vi "HSOpMux.vi"() -> ()   [LabVIEW 2013]
uses:
  Multiplexer_Opmux.lvclass
  HS3.llb/GlobalVariables.vi
  OverallRoutines/HS3OverallRoutines.lvlib
panel:
  in  "TimeForEachScan":dbl[](array[numeric])
  out "tmr":u32 caption="Elapsed for acq"
  in  "Run":bool
  out "Channels":refnum<vi>[](array[refnum])
  out "Ch8":dbl[](graph)
  out "Ch7":dbl[](graph)
  out "Ch6":dbl[](graph)
  out "Ch5":dbl[](graph)
  out "Ch4":dbl[](graph)
  out "Ch3":dbl[](graph)
  out "Ch2":dbl[](graph)
  out "Ch1":dbl[](graph)
  in  "Scan":bool
  in  "Set":bool
  in  "Length":dbl=1.0 caption="Length (us)" min=0.1 max=6.3 step=0.1
  in  "Voltage":dbl min=0.0 max=1023.0 step=1.0
  in  "Into":u16[](array[numeric])
  in  "Forward":u16[](array[numeric])
  in  "Signal Frequency":u32(ring)=10000000 items=["5Mhz"=5000000, "10Mhz"=10000000, "25Mhz"=25000000]
  in  "Shutdown":bool
  out "Acq":bool caption="Acquiring"
  out "SampleFrequency":dbl format="%#_8g"
  out "ChArray":dbl[](array[numeric])
  out "Serial":i32
  out "DllPath":path
  out "HandyScope":bool
  out "Multiplexer":bool
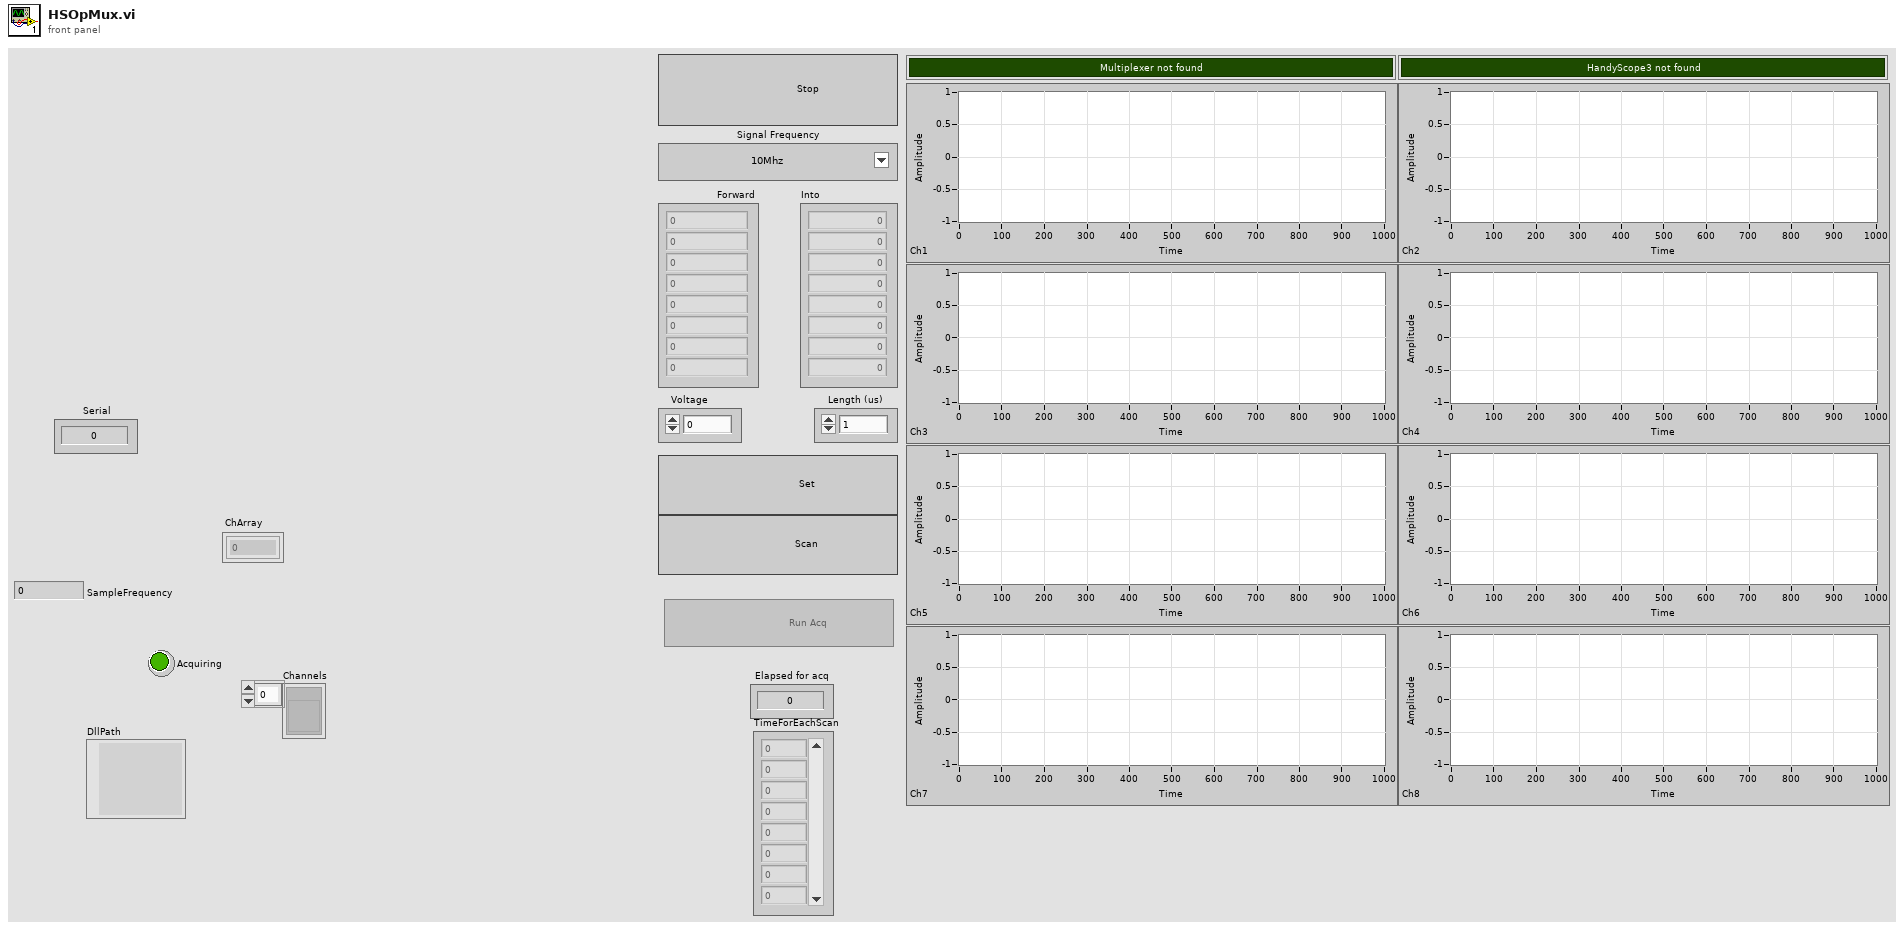
[diagram p1: front panel]
types:
  T1 = cluster{"trgSource":u16, "trgMode":u16, "trgLevel":dbl}
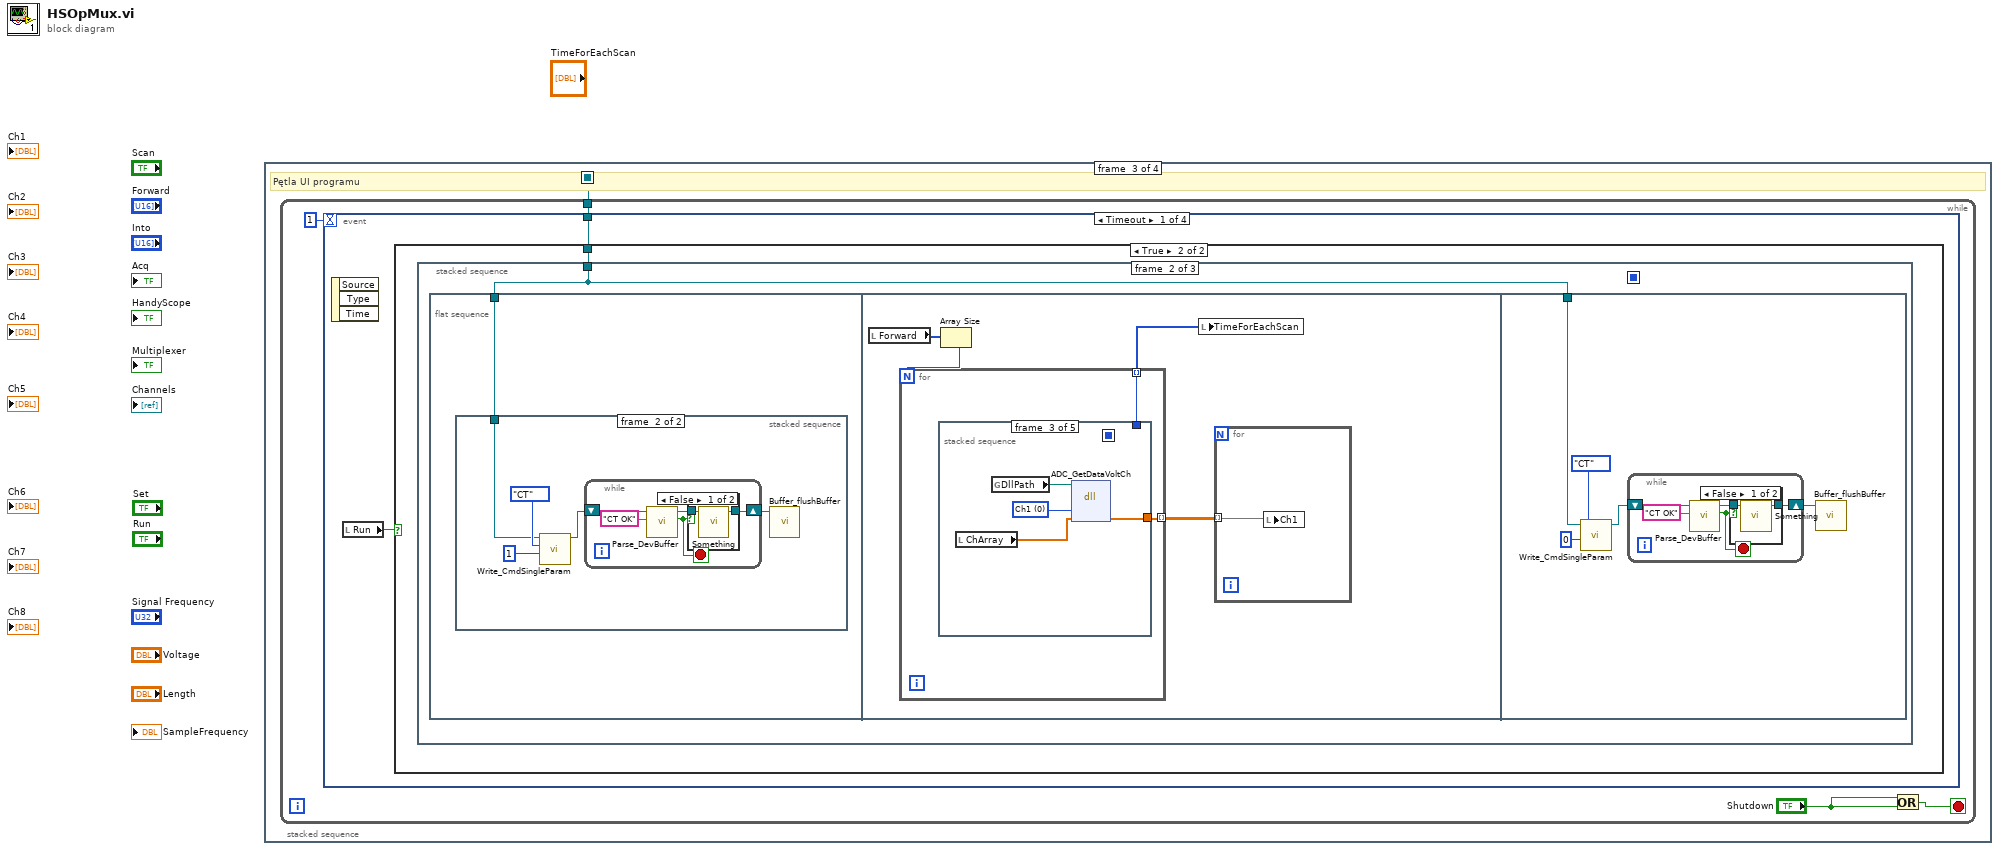
[diagram p0: block diagram]
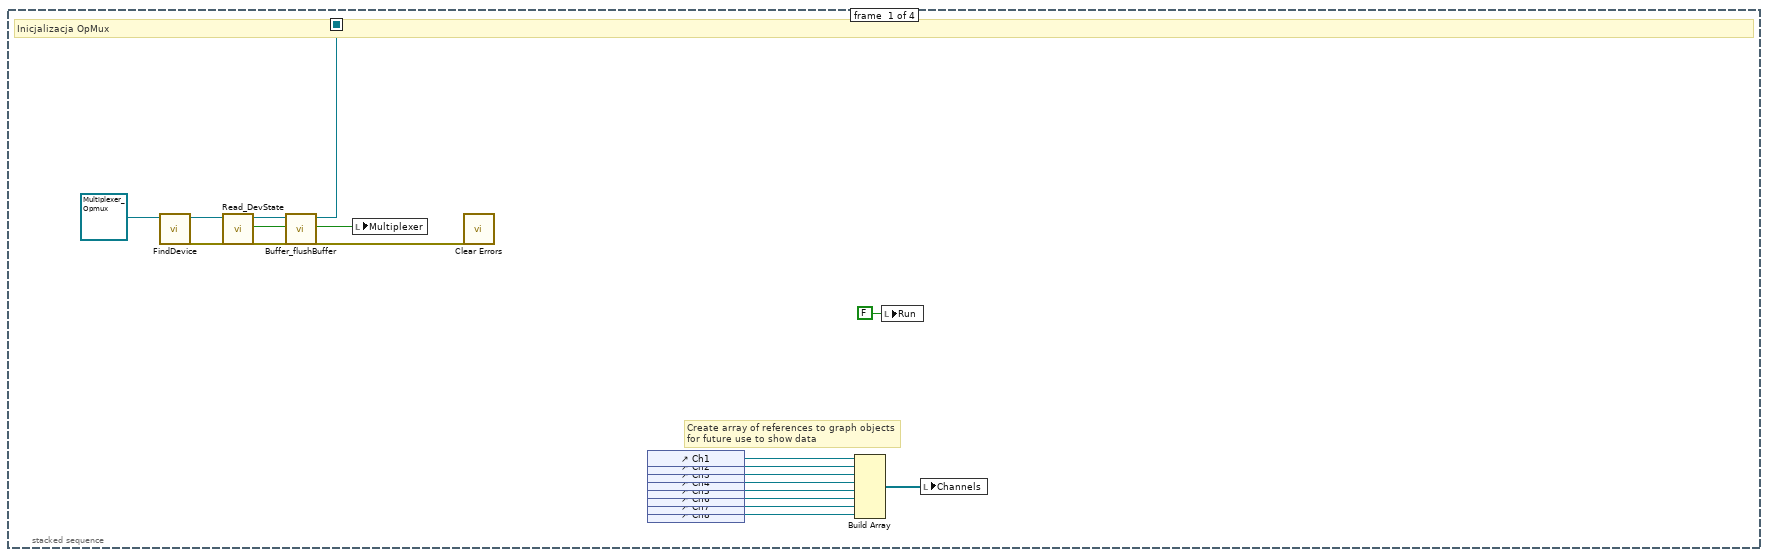
[diagram p2: hidden frame]
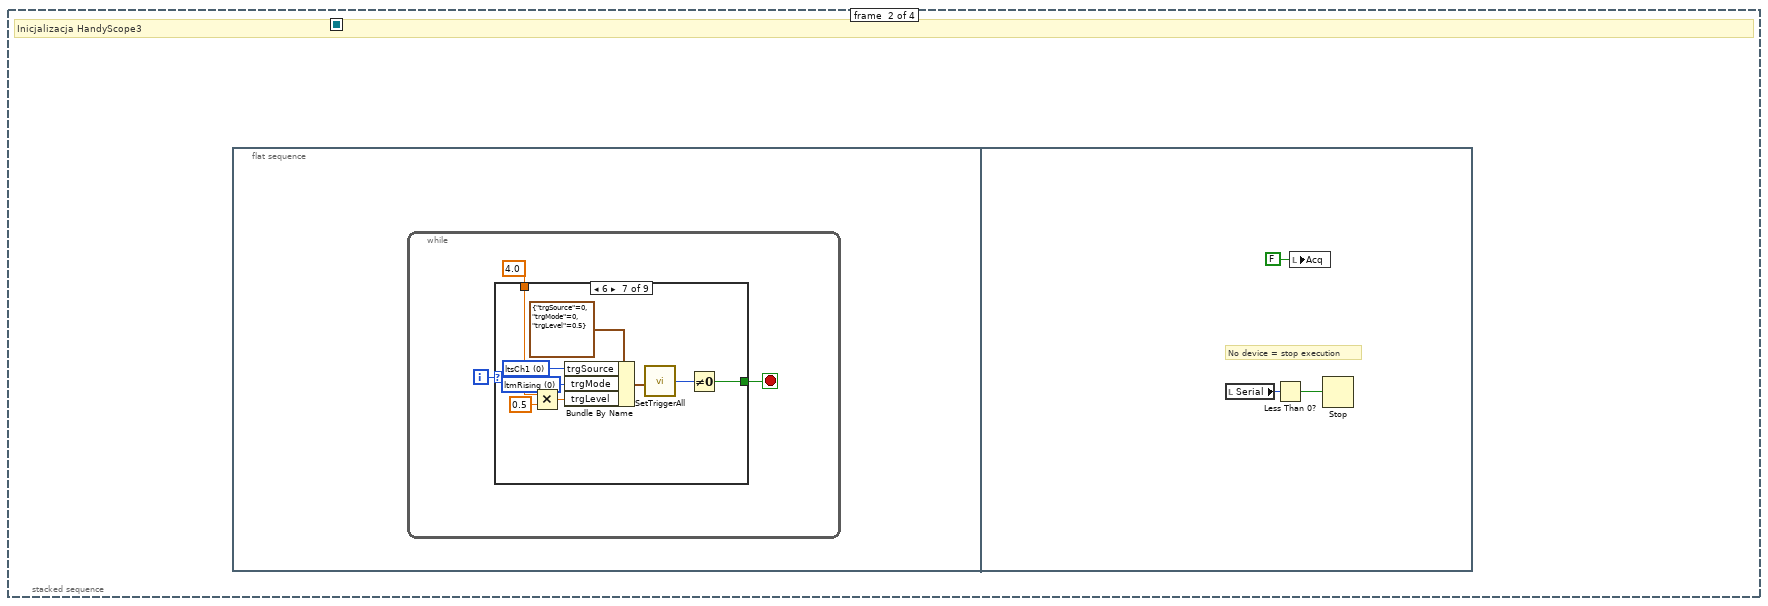
[diagram p3: hidden frame]
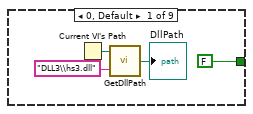
[diagram p4: hidden frame]
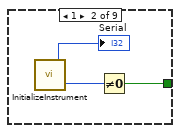
[diagram p5: hidden frame]
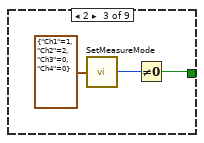
[diagram p6: hidden frame]
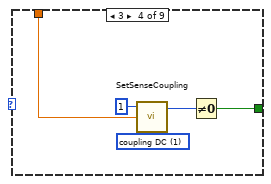
[diagram p7: hidden frame]
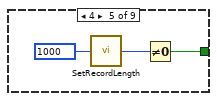
[diagram p8: hidden frame]
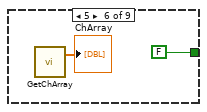
[diagram p9: hidden frame]
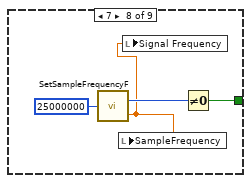
[diagram p10: hidden frame]
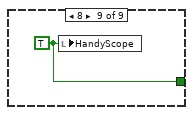
[diagram p11: hidden frame]
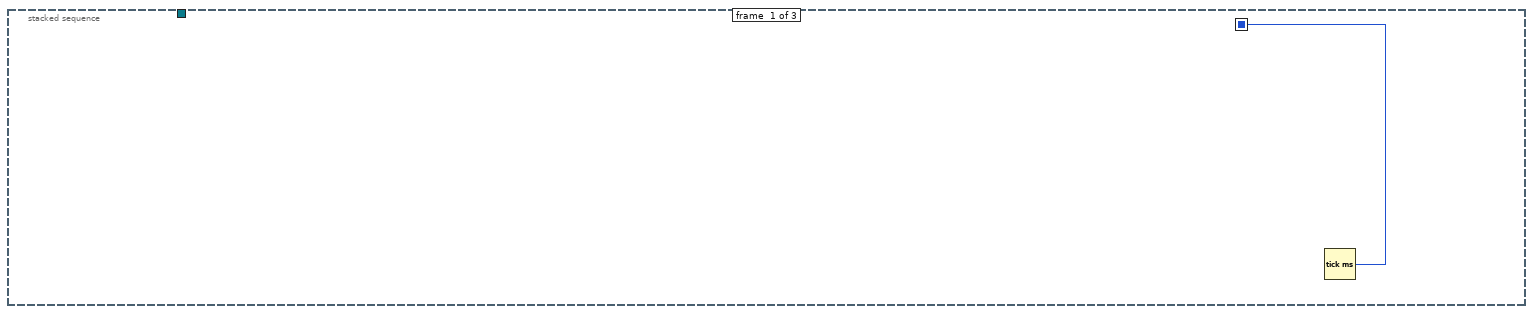
[diagram p13: hidden frame]
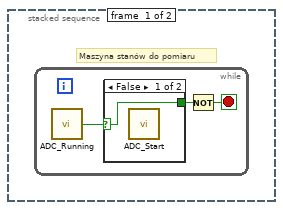
[diagram p14: hidden frame]
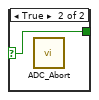
[diagram p15: hidden frame]
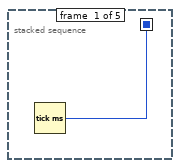
[diagram p17: hidden frame]
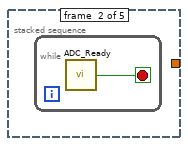
[diagram p18: hidden frame]
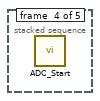
[diagram p19: hidden frame]
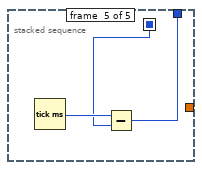
[diagram p20: hidden frame]
diagram:
  n1 = stacked-sequence {
    seq-local: [w1 _ _ _] -> [_ _ w59 _]
    frame #0 {
      # "Create array of references to graph objects\nfor future use to show data"
      # "Inicjalizacja OpMux"
      n2 = call-dynamic "FindDevice.vi"("Multiplexer_Opmux in"=refnum<class "Multiplexer_Opmux.lvclass"> refnum) -> ("error out"=w15:errorcluster, "Multiplexer_Opmux out"=w17:refnum<class "Multiplexer_Opmux.lvclass">)  [unwired: 8 in, 1 out]
      n3 = call-dynamic "Read_DevState.vi"("error in (no error)"=w15, "Multiplexer_Opmux in"=w17) -> ("error out"=w3:errorcluster, "DevState"=w16:bool, "Multiplexer_Opmux out"=w4:refnum<class "Multiplexer_Opmux.lvclass">)  [unwired: 7 in]
      n4 = call-dynamic "Buffer_flushBuffer.vi"("error in (no error)"=w3, "Multiplexer_Opmux in"=w4) -> ("error out"=w2:errorcluster, "Multiplexer_Opmux out"=w1:refnum<class "Multiplexer_Opmux.lvclass">)  [unwired: 8 in]
      n5 = local write "Multiplexer"(w16) -> ()
      n6 = call <vilib>:"Clear Errors.vi"("error in (no error)"=w2) -> ()  [unwired: 6 in, 1 out]
      n7 = control-ref of="Ch1"() -> (w14:refnum<vi>)
      n8 = control-ref of="Ch2"() -> (w13:refnum<vi>)
      n9 = control-ref of="Ch3"() -> (w12:refnum<vi>)
      n10 = control-ref of="Ch4"() -> (w11:refnum<vi>)
      n11 = control-ref of="Ch5"() -> (w10:refnum<vi>)
      n12 = control-ref of="Ch6"() -> (w9:refnum<vi>)
      n13 = control-ref of="Ch7"() -> (w8:refnum<vi>)
      n14 = control-ref of="Ch8"() -> (w7:refnum<vi>)
      n15 = Build Array(w14, w13, w12, w11, w10, w9, w8, w7) -> (w6:refnum<vi>[])
      n16 = local write "Run"(FALSE ("Run")) -> ()
      n17 = local write "Channels"(w6) -> ()
    }
    frame #1 {
      # "Inicjalizacja HandyScope3"
      n18 = flat-sequence {
        frame #0 {
          n19 = while {
            i -> [w21]
            stop <- w20 stop-if-true
            w19 = 4.0 items=["0,2"=0.2, "0,8"=0.8, "2"=2.0, "4"=4.0, "20"=20.0, "40"=40.0, "80"=80.0] ("chSense")
            n20 = case shown="6" w21 {
              tunnel: [FALSE w26 w30 w33 w38 FALSE w49 w54 w55] -> w20
              tunnel: w19 -> [_ _ _ w32 _ _ w45 _ _]
              frame 0, Default {
                n21 = Current VI's Path() -> (path=w23:path)
                n22 = call "GetDllPath.vi"("DllName"="DLL3\\hs3.dll", "path"=w23) -> ("DllPath"=→"DllPath":path)
              }
              frame 1 {
                n23 = call "InitializeInstrument.vi"() -> ("ErrorCode"=w27:i16, "Serial"=→"Serial":i32)
                n24 = Not Equal To 0?(x=w27) -> (x != 0?=w26:bool)
              }
              frame 2 {
                n25 = call "SetMeasureMode.vi"("oModeStack"=cluster{"Ch1":u8, "Ch2":u8, "Ch3":u8, "Ch4":u8} {"Ch1"=1, "Ch2"=2, "Ch3"=0, "Ch4"=0}) -> ("ErrorCode"=w29:i16)
                n26 = Not Equal To 0?(x=w29) -> (x != 0?=w30:bool)
              }
              frame 3 {
                w36 = 1 items=["coupling AC", "coupling DC"] ("chCoupling")
                n27 = call "SetSenseCoupling.vi"("chCoupling"=w36, "chSense"=w32, "chSet"=1) -> ("ErrorCode"=w34:i16)  [unwired: 1 out]
                n28 = Not Equal To 0?(x=w34) -> (x != 0?=w33:bool)
              }
              frame 4 {
                w39 = u32 1000 items=["100"=100, "250"=250, "500"=500, "1000"=1000, "2500"=2500, "5000"=5000, "10000"=10000, "25000"=25000, "50000"=50000, "100000"=100000, "131000"=131000] ("RecordLength")
                n29 = call "SetRecordLength.vi"("RecordLength"=w39) -> ("ErrorCode"=w37:i16)
                n30 = Not Equal To 0?(x=w37) -> (x != 0?=w38:bool)
              }
              frame 5 {
                n31 = call "GetChArray.vi"() -> ("ChArray"=→"ChArray":dbl[])  [unwired: 1 out]
              }
              frame 6 {
                w42 = u16 0 items=["ltmRising", "ltmFalling", "ltmInWindow", "ltmOutWindow", "ltmTVLine", "ltmTVFieldOdd", "ltmTVFieldEven"] ("trgMode")
                w43 = u16 0 items=["ltsCh1"=0, "ltsCh2"=1, "ltsExternal"=4, "ltsAnalogExt"=5, "ltsAnd"=6, "ltsOr"=7, "ltsXor"=8, "ltsNoTrig"=9, "notUsed"=10, "ltsPxiExt"=11, "ltsGenStart"=12, "ltsGenStop"=13, "ltsGenNew"=14] ("trgSource")
                n32 = Multiply(x=w45, y=0.5) -> (x*y=w46:dbl)
                n33 = Bundle By Name(cluster=T1 {"trgSource"=0, "trgMode"=0, "trgLevel"=0.5} ("TriggerSettings"), "trgSource"=w43, "trgMode"=w42, "trgLevel"=w46) -> (w47:T1)
                n34 = call "SetTriggerAll.vi"("TriggerSettings"=w47) -> ("ErrorCode"=w50:i32)
                n35 = Not Equal To 0?(x=w50) -> (x != 0?=w49:bool)
              }
              frame 7 {
                n36 = call "SetSampleFrequencyF.vi"("Numeric Control"=u32 25000000) -> ("ErrorCode"=w53:i16, "oFreq_Set"=w52:dbl)
                n37 = local write "SampleFrequency"(w52) -> ()
                n38 = local write "Signal Frequency"(w52) -> ()
                n39 = Not Equal To 0?(x=w53) -> (x != 0?=w54:bool)
              }
              frame 8 {
                w55 = TRUE ("HandyScope")
                n40 = local write "HandyScope"(w55) -> ()
              }
            }
          }
        }
        frame #1 {
          # "No device = stop execution"
          n41 = local read "Serial"() -> (w58:i32)
          n42 = Less Than 0?(x=w58) -> (x < 0?=w57:bool)
          n43 = local write "Acq"(FALSE ("Acq")) -> ()
          n44 = Stop(stop? (T)=w57) -> ()
        }
      }
    }
    frame #2 {
      # "Pętla UI programu"
      n45 = while {
        tunnel: w59 -> [w60]
        stop <- w62 stop-if-true
        n46 = event shown="[0] Timeout" {
          selector: _ -> [_ _ _ _]
          dyn-events: _ -> [_ _ _ _]
          timeout: 1 -> [_ _ _ _]
          tunnel: w60 -> [w65 _ w121 _]
          event Timeout {
            n47 = event-data() -> ()  [unwired: 1 in, 3 out]
            n48 = local read "Run"() -> (w64:bool)
            n49 = case shown="True" w64 {
              tunnel: w65 -> [_ w66]
              frame False {
              }
              frame True {
                n50 = stacked-sequence {
                  seq-local: [w67 _ _] -> [_ _ w118]
                  tunnel: w66 -> [_ w68 _]
                  frame #0 {
                    n51 = Tick Count (ms)() -> (millisecond timer value=w67:u32)
                  }
                  frame #1 {
                    n52 = flat-sequence {
                      tunnel: w68 -> [w69]
                      tunnel: w68 -> [w106]
                      frame #0 {
                        n53 = stacked-sequence {
                          tunnel: w69 -> [_ w75]
                          frame #0 {
                            # "Maszyna stanów do pomiaru"
                            n54 = while {
                              stop <- w71 stop-if-true
                              n55 = call "ADC_Running.vi"() -> ("Measuring"=w72:bool)
                              n56 = case shown="False" w72 {
                                selector: w72 -> [w73 w74]
                                tunnel: [w73 w74] -> w70
                                frame False {
                                n57 = call "ADC_Start.vi"() -> ()  [unwired: 1 out]
                                }
                                frame True {
                                n58 = call "ADC_Abort.vi"() -> ()  [unwired: 1 out]
                                }
                              }
                              n59 = Not(x=w70) -> (.not. x?=w71:bool)
                            }
                          }
                          frame #1 {
                            n60 = call-dynamic "Write_CmdSingleParam.vi"("Param"=1, "Command"=enum16{"SA", "GT", "SI", "SL", "ST", "CT"}."CT", "Multiplexer_Opmux in"=w75) -> ("Multiplexer_Opmux out"=w77:refnum<class "Multiplexer_Opmux.lvclass">)  [unwired: 7 in, 1 out]
                            n61 = while {
                              shift-right: [w81] -> w76
                              shift-left: w77 -> [w80]
                              stop <- w83 stop-if-true
                              n62 = call-dynamic "Parse_DevBuffer.vi"("searchFor"="CT OK", "Multiplexer_Opmux in"=w80) -> ("Found"=w83:bool, "Multiplexer_Opmux out"=w84:refnum<class "Multiplexer_Opmux.lvclass">)  [unwired: 7 in, 1 out]
                              n63 = case shown="False" w83 {
                                tunnel: w84 -> [w86 w87]
                                tunnel: [w85 w87] -> w81
                                frame False {
                                n64 = call-dynamic "Something.vi"("Multiplexer_Opmux in"=w86) -> ("Multiplexer_Opmux out"=w85:refnum<class "Multiplexer_Opmux.lvclass">)  [unwired: 9 in, 1 out]
                                }
                                frame True {
                                }
                              }
                            }
                            n65 = call-dynamic "Buffer_flushBuffer.vi"("Multiplexer_Opmux in"=w76) -> ()  [unwired: 9 in, 2 out]
                          }
                        }
                      }
                      frame #1 {
                        n66 = local read "Forward"() -> (w91:u16[])
                        n67 = Array Size(array=w91) -> (size(s)=w90:i32)
                        n68 = for {
                          N: w90 -> [_]
                          tunnel: [w94] -> w89 mode=indexing
                          tunnel: [w93] -> w88 mode=indexing
                          n69 = stacked-sequence {
                            seq-local: [w95 _ _ _ _] -> [_ _ _ _ w102]
                            tunnel: [_ _ _ _ w101] -> w94
                            tunnel: [_ _ w97 _ _] -> w93
                            frame #0 {
                              n70 = Tick Count (ms)() -> (millisecond timer value=w95:u32)
                            }
                            frame #1 {
                              n71 = while {
                                stop <- w96 stop-if-true
                                n72 = call "ADC_Ready.vi"() -> ("Ready"=w96:bool)
                              }
                            }
                            frame #2 {
                              w100 = u8 0 items=["Ch1", "Ch2", "Ch3", "Ch4"] ("Ch")
                              n73 = local read "ChArray"() -> (w98:dbl[])
                              n74 = global read "GlobalVariables.vi" "DllPath"() -> (w99:path)
                              n75 = dll-call lib="?" fn="ADC_GetDataVoltCh"(path in=w99, "Ch"=w100, "chData"=w98) -> ("chData"=w97:dbl[])  [unwired: 4 in, 2 out]
                            }
                            frame #3 {
                              n76 = call "ADC_Start.vi"() -> ()  [unwired: 1 out]
                            }
                            frame #4 {
                              n77 = Tick Count (ms)() -> (millisecond timer value=w103:u32)
                              n78 = Subtract(x=w103, y=w102) -> (x-y=w101:u32)
                            }
                          }
                        }
                        n79 = local write "TimeForEachScan"(w89) -> ()
                        n80 = for {
                          tunnel: w88 -> [w92] mode=indexing
                          n81 = local write "Ch1"(w92) -> ()
                        }
                      }
                      frame #2 {
                        n82 = call-dynamic "Write_CmdSingleParam.vi"("Param"=0, "Command"=enum16{"SA", "GT", "SI", "SL", "ST", "CT"}."CT", "Multiplexer_Opmux in"=w106) -> ("Multiplexer_Opmux out"=w105:refnum<class "Multiplexer_Opmux.lvclass">)  [unwired: 7 in, 1 out]
                        n83 = while {
                          shift-right: [w110] -> w104
                          shift-left: w105 -> [w109]
                          stop <- w112 stop-if-true
                          n84 = call-dynamic "Parse_DevBuffer.vi"("searchFor"="CT OK", "Multiplexer_Opmux in"=w109) -> ("Found"=w112:bool, "Multiplexer_Opmux out"=w113:refnum<class "Multiplexer_Opmux.lvclass">)  [unwired: 7 in, 1 out]
                          n85 = case shown="False" w112 {
                            tunnel: w113 -> [w115 w116]
                            tunnel: [w114 w116] -> w110
                            frame False {
                              n86 = call-dynamic "Something.vi"("Multiplexer_Opmux in"=w115) -> ("Multiplexer_Opmux out"=w114:refnum<class "Multiplexer_Opmux.lvclass">)  [unwired: 9 in, 1 out]
                            }
                            frame True {
                            }
                          }
                        }
                        n87 = call-dynamic "Buffer_flushBuffer.vi"("Multiplexer_Opmux in"=w104) -> ()  [unwired: 9 in, 2 out]
                      }
                    }
                  }
                  frame #2 {
                    n88 = Tick Count (ms)() -> (millisecond timer value=w119:u32)
                    n89 = Subtract(x=w119, y=w118) -> (x-y=→"tmr":u32)
                  }
                }
              }
            }
          }
          event "Scan": Value Change {
            n90 = event-data() -> ()  [unwired: 1 in, 6 out]
          }
          event "Set": Value Change {
            n91 = event-data() -> ()  [unwired: 1 in, 6 out]
            n92 = local write "Set"(FALSE ("Set")) -> ()
            n93 = stacked-sequence {
              tunnel: w121 -> [w124 _ w126 _ w131 _ w137 _ w141 _ w143]
              frame #0 {
                n94 = call-dynamic "Write_CmdSingleParam.vi"("Param"=0, "Command"=enum16{"SA", "GT", "SI", "SL", "ST", "CT"}."CT", "Multiplexer_Opmux in"=w124) -> ()  [unwired: 7 in, 2 out]
                n95 = call "ADC_Abort.vi"() -> ()  [unwired: 1 out]
              }
              frame #1 {
                n96 = Wait (ms)(milliseconds to wait=u32 50) -> ()  [unwired: 1 out]
              }
              frame #2 {
                n97 = local read "Forward"() -> (w129:u16[])
                n98 = local read "Into"() -> (w128:u16[])
                n99 = call-dynamic "Write_CmdMultipleParam.vi"("Command"=enum16{"ST"}."ST", "Table2"=w128, "Table1"=w129, "Multiplexer_Opmux in"=w126) -> ()  [unwired: 6 in, 2 out]
              }
              frame #3 {
                n100 = Wait (ms)(milliseconds to wait=u32 50) -> ()  [unwired: 1 out]
              }
              frame #4 {
                n101 = local read "Length"() -> (w133:dbl)
                n102 = Multiply(x=w133, y=10.0) -> (x*y=w134:dbl)
                n103 = call-dynamic "Write_CmdSingleParam.vi"("Param"=w134, "Command"=enum16{"SA", "GT", "SI", "SL", "ST", "CT"}."SL", "Multiplexer_Opmux in"=w131) -> ()  [unwired: 7 in, 2 out]
              }
              frame #5 {
                n104 = Wait (ms)(milliseconds to wait=u32 50) -> ()  [unwired: 1 out]
              }
              frame #6 {
                n105 = local read "Voltage"() -> (w139:dbl)
                n106 = call-dynamic "Write_CmdSingleParam.vi"("Param"=w139, "Command"=enum16{"SA", "GT", "SI", "SL", "ST", "CT"}."SI", "Multiplexer_Opmux in"=w137) -> ()  [unwired: 7 in, 2 out]
              }
              frame #7 {
                n107 = Wait (ms)(milliseconds to wait=u32 50) -> ()  [unwired: 1 out]
              }
              frame #8 {
                n108 = call-dynamic "Buffer_flushBuffer.vi"("Multiplexer_Opmux in"=w141) -> ()  [unwired: 9 in, 2 out]
              }
              frame #9 {
                n109 = Wait (ms)(milliseconds to wait=u32 25) -> ()  [unwired: 1 out]
              }
              frame #10 {
                n110 = local write "Run"(TRUE ("Run")) -> ()
                n111 = call-dynamic "Write_CmdSingleParam.vi"("Param"=1, "Command"=enum16{"SA", "GT", "SI", "SL", "ST", "CT"}."CT", "Multiplexer_Opmux in"=w143) -> ()  [unwired: 7 in, 2 out]
              }
            }
          }
          event "Signal Frequency": Value Change {
            n112 = event-data() -> ("NewVal"=w147:u32)  [unwired: 1 in, 5 out]
            n113 = stacked-sequence {
              tunnel: w147 -> [w151 _]
              frame #0 {
                n114 = call "SetSampleFrequencyF.vi"("Numeric Control"=w151) -> ("ErrorCode"=w150:i16, "oFreq_Set"=w149:dbl)
                n115 = case shown="True" TRUE {
                  tunnel: w149 -> [_ w155]
                  frame False {
                  }
                  frame True {
                    # "Do 100us sygnał zmieniamy automatycznie"
                    n116 = Multiply(x=w155, y=4e-05) -> (x*y=w153:dbl)
                    n117 = To Unsigned Long Integer(number=w153) -> (unsigned 32bit integer=w154:u32)
                    n118 = call "SetRecordLength.vi"("RecordLength"=w154) -> ()  [unwired: 1 out]
                  }
                }
                n119 = local write "SampleFrequency"(w149) -> ()
                n120 = call "Error Converter (ErrCode or Status).vi"("error code"=w150) -> ()  [unwired: 10 in, 1 out]
              }
              frame #1 {
              }
            }
          }
        }
        n121 = Or(x="Shutdown", y="Shutdown") -> (x .or. y?=w62:bool)
      }
    }
    frame #3 {
      # "Rozłączenie urządzeń po zakończeniu działania programu"
    }
  }
